vi "daqio_Create_or_Update_Tag.vi"(6 "Tag Data Type (create-only)":string(combo)="string", 8 "error in (no error)":errorcluster, 9 "Tag Value":string, 10 "Tag Key":string, 11 "daq.io type in":T1={"daq.io ref"=refnum, "daq.io API Base"="http://dashboard.daq.io/api/v1", "Device Key"="", "Account ID"="", "online"=TRUE, "SSL"=FALSE, "buffer"=TRUE}) -> (0 "error out":errorcluster, 2 "JSON string":string, 3 "daq.io type out":T1={"daq.io ref"=refnum, "daq.io API Base"="http://dashboard.daq.io/api/v1", "Device Key"="", "Account ID"="", "online"=TRUE, "SSL"=FALSE, "buffer"=TRUE})   [LabVIEW 2013, in "daqio minimal.lvlib"]
doc: "This VI will update or create a Tag for a specific Device on daq.io. \nIt will search the Tags on the device and either update or create it. In order to create it, it will define a new Tag for the Device."
uses:
  daqio minimal.lvlib
  _typedefs/daqio-Type.ctl
  <vilib>/httpClient/ClientHandle.ctl
  _typedefs/daqio-Device-Tags.ctl
  _typedefs/daqio-Device-Just-Tags.ctl
  <vilib>/Easy HTTP Client/Easy HTTP.lvlib
  <vilib>/httpClient/LabVIEWHTTPClient.lvlib
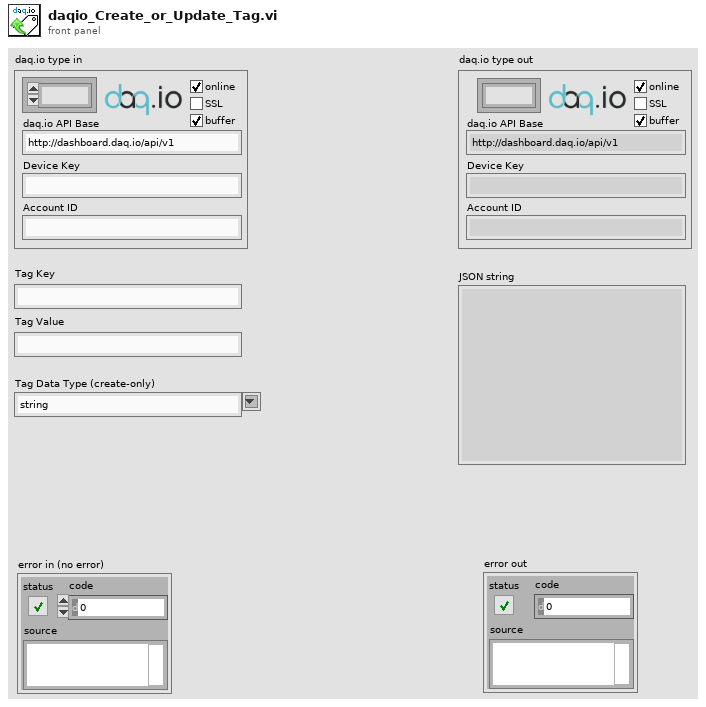
[diagram p1: front panel]
types:
  T1 = typedef "daqio minimal.lvlib/daqio-Type.ctl" = cluster{"daq.io ref":T2, "daq.io API Base":string, "Device Key":string, "Account ID":string, "online":bool, "SSL":bool, "buffer":bool}
  T2 = typedef "LabVIEWHTTPClient.lvlib/ClientHandle.ctl" = refnum<k1>
  T3 = typedef "daqio minimal.lvlib/daqio-Device-Just-Tags.ctl" = cluster{"tags":cluster{"key":string, "value":string}[]}
  T4 = typedef "daqio minimal.lvlib/daqio-Device-Tags.ctl" = cluster{"key":string, "value":string}[]
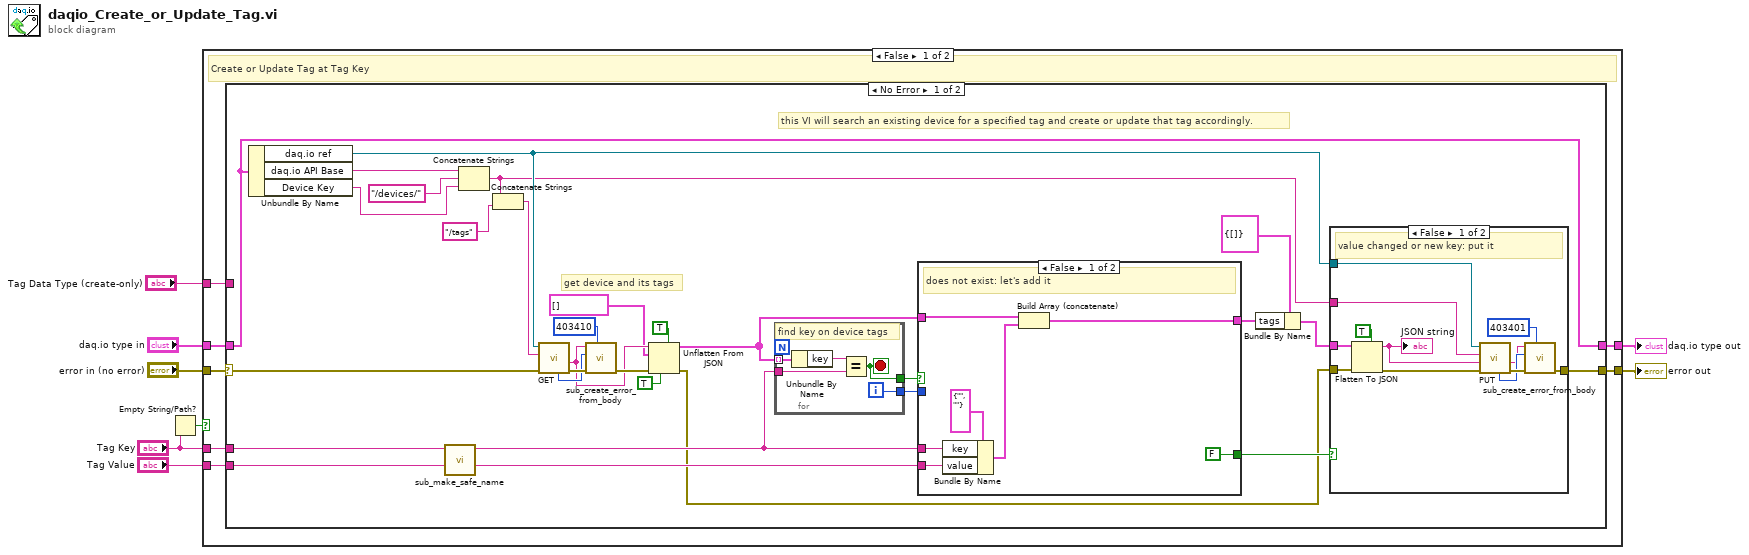
[diagram p0: block diagram]
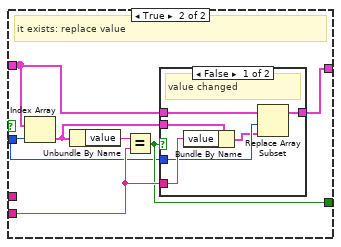
[diagram p2: hidden frame]
diagram:
  n1 = Empty String/Path?(string/path="Tag Key") -> (empty?=w2:bool)
  n2 = case shown="False" w2 {
    tunnel: "error in (no error)" -> [w15 w86]
    tunnel: "daq.io type in" -> [w14 w87]
    tunnel: [w13 w86] -> w6
    tunnel: [w12 w87] -> w5
    tunnel: "Tag Value" -> [w11 _]
    tunnel: "Tag Key" -> [w10 _]
    tunnel: "Tag Data Type (create-only)" -> [w9 _]
    frame False {
      # "Create or Update Tag at Tag Key"
      n3 = case shown="No Error" w15 {
        selector: w15 -> [w37 w85]
        tunnel: w14 -> [w23 w84]
        tunnel: [w44 w85] -> w13
        tunnel: [w23 w84] -> w12
        tunnel: w11 -> [w42 _]
        tunnel: w10 -> [w41 _]
        tunnel: w9 -> [_ _]
        frame No Error {
          # "get device and its tags"
          # "this VI will search an existing device for a specified tag and create or update that tag accordingly."
          n4 = Unbundle By Name(w23) -> ("daq.io ref"=w38:T2, "daq.io API Base"=w43:string, "Device Key"=w33:string)
          n5 = call "sub_make_safe_name.vi"("Input String"=w41) -> ("Safe Output String"=w27:string)  [unwired: 10 in]
          n6 = Concatenate Strings(w43, "/devices/", w33) -> (w18:string)
          n7 = Concatenate Strings(w18, "/tags" ("string")) -> (w17:string)
          n8 = call <vilib>:"GET.vi"("error in (no error)"=w37, "url"=w17, "client handle"=w38) -> ("error out"=w36:errorcluster, "body"=w31:string, "HTTP Response Code"=w35:i32)  [unwired: 4 in, 2 out]
          n9 = call "sub_create_error_from_body.vi"("error code"=403410, "error in (no error)"=w36, "http code"=w35, "body"=w31) -> ("error out"=w32:errorcluster)  [unwired: 7 in]
          n10 = Unflatten From JSON(enable LabVIEW extensions? (T)=TRUE, JSON string=w31, type and defaults=T4 [] ("tags"), default null elements? (F)=TRUE, error in (no error)=w32) -> (value=w20:T4, error out=w25:errorcluster)  [unwired: 2 in]
          n11 = for {
            tunnel: w27 -> [w70]
            tunnel: [w69] -> w29
            tunnel: w20 -> [w68] mode=indexing
            tunnel: [w66] -> w28
            i -> [w69]
            stop <- w66 stop-if-true
            # "find key on device tags"
            n12 = Unbundle By Name(w68) -> ("key"=w67:string)
            n13 = Equal?(x=w67, y=w70) -> (x = y?=w66:bool)
          }
          n14 = case shown="False" w28 {
            tunnel: w42 -> [w49 w58]
            tunnel: [FALSE w57] -> w40
            tunnel: w20 -> [w51 w56]
            tunnel: w29 -> [_ w55]
            tunnel: w27 -> [w48 _]
            tunnel: [w46 w52] -> w26
            frame False {
              # "does not exist: let's add it"
              n15 = Bundle By Name(cluster=cluster{"key":string, "value":string} {"key"="", "value"=""} ("Cluster"), "key"=w48, "value"=w49) -> (w47:cluster{"key":string, "value":string})
              n16 = Build Array (concatenate)(w51, w47) -> (w46:T4)
            }
            frame True {
              # "it exists: replace value"
              n17 = Index Array(array=w56, index=w55) -> (element=w53:cluster{"key":string, "value":string})
              n18 = Unbundle By Name(w53) -> ("value"=w54:string)
              n19 = Equal?(x=w54, y=w58) -> (x = y?=w57:bool)
              n20 = case shown="False" w57 {
                tunnel: w58 -> [w64 _]
                tunnel: w55 -> [w63 _]
                tunnel: w56 -> [w61 w65]
                tunnel: w53 -> [w60 _]
                tunnel: [w59 w65] -> w52
                frame False {
                  # "value changed"
                  n21 = Bundle By Name(cluster=w60, "value"=w64) -> (w62:cluster{"key":string, "value":string})
                  n22 = Replace Array Subset(array=w61, new element=w62, index=w63) -> (w59:T4)
                }
                frame True {
                  # "same value"
                }
              }
            }
          }
          n23 = Bundle By Name(cluster=T3 {"tags"=[]} ("Device"), "tags"=w26) -> (w24:T3)
          n24 = case shown="False" w40 {
            tunnel: [w81 w83] -> w44
            tunnel: w38 -> [w79 _]
            tunnel: w25 -> [w73 w83]
            tunnel: w24 -> [w72 _]
            tunnel: w18 -> [w71 _]
            frame False {
              # "value changed or new key: put it"
              n25 = Flatten To JSON(enable LabVIEW extensions? (T)=TRUE, anything=w72, error in (no error)=w73) -> (JSON string=w77:string, 11:w76:errorcluster)
              "JSON string" <- w77
              n26 = call <vilib>:"PUT.vi"("error in (no error)"=w76, "data"=w77, "url"=w71, "client handle"=w79) -> ("error out"=w82:errorcluster, "body"=w74:string, "HTTP Response Code"=w80:i32)  [unwired: 3 in, 2 out]
              n27 = call "sub_create_error_from_body.vi"("error code"=403401, "error in (no error)"=w82, "http code"=w80, "body"=w74) -> ("error out"=w81:errorcluster)  [unwired: 7 in]
            }
            frame True {
              # "same value, does not need to be updated"
            }
          }
        }
        frame Error {
        }
      }
    }
    frame True {
    }
  }
  "error out" <- w6
  "daq.io type out" <- w5
